vi "csvFormatter.vi"(5 "Sensor Data In":string, 7 "Iteration":u32, 10 "error in (no error)":errorcluster) -> (2 "error out":errorcluster, 3 "CSV formatted String":string)   [LabVIEW 2018]
panel:
  in  "error in (no error) 2":errorcluster
  out "error out 2":errorcluster
  in  "Iteration 2":u32
  in  "Sensor Data In 2":string
  out "CSV formatted String 2":string
  # "FITS Table Requirement:\n1> Detector ID (either 1 or 2)\n2> Pixel ID (0 - 256)\n3> PHA (Energy Value)\n4> Time Stamp (Clk count)\n5?  CZT Tick Count"
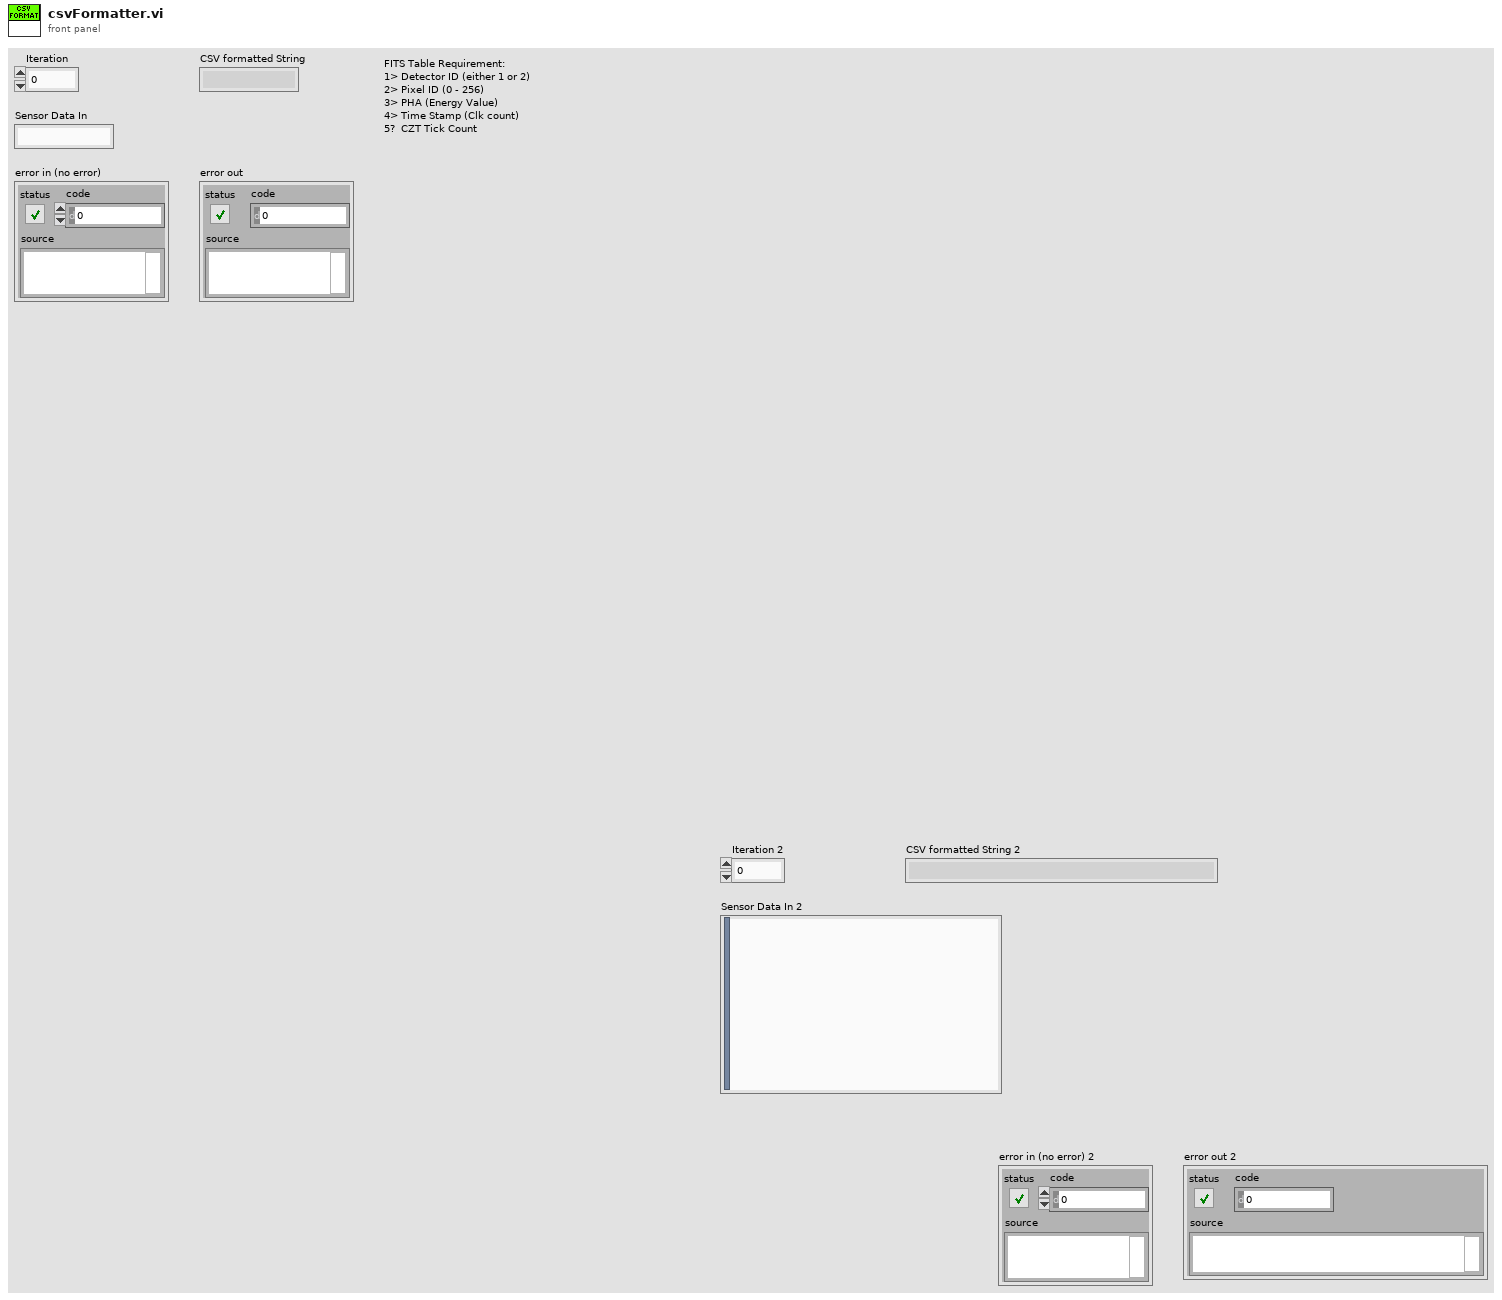
[diagram p1: front panel]
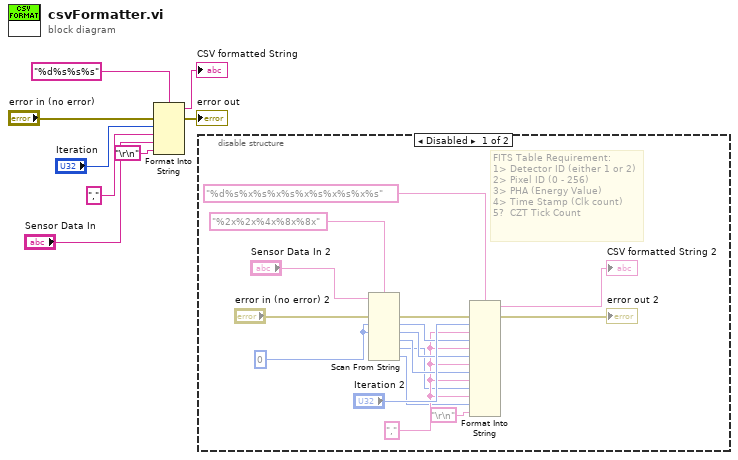
[diagram p0: block diagram]
diagram:
  n1 = Format Into String(format string="%d%s%s%s", error in="error in (no error)", "Iteration", "," ("Column separator"), "Sensor Data In", "\r\n" ("row separator")) -> (resulting string=→"CSV formatted String":string, error out=→"error out":errorcluster)  [unwired: 1 in]
  n2 = disable-structure shown="Disabled" {
    frame Disabled {
      w9 = u16 0
      w13 = "," ("Column separator")
      # "FITS Table Requirement:\n1> Detector ID (either 1 or 2)\n2> Pixel ID (0 - 256)\n3> PHA (Energy Value)\n4> Time Stamp (Clk count)\n5?  CZT Tick Count"
      n3 = Scan From String(format string="%2x%2x%4x%8x%8x", input string="Sensor Data In 2", error in="error in (no error) 2", default 1=w9, default 2=w9) -> (error out=w17:errorcluster, output 1=w16:u16, output 2=w15:u16, output 3=w14:u32, output 4=w12:u32, output 5=w11:u32)  [unwired: 4 in, 2 out]
      n4 = Format Into String(format string="%d%s%x%s%x%s%x%s%x%s%x%s", error in=w17, "Iteration 2", w13, w16, w13, w15, w13, w14, w13, w12, w13, w11, "\r\n" ("row separator")) -> (resulting string=→"CSV formatted String 2":string, error out=→"error out 2":errorcluster)  [unwired: 1 in]
    }
    frame Enabled {
    }
  }
